vi "Valiadate Plugin Name.vi"(0 "Path":path, 5 "library name":string, 11 "error in (no error)":errorcluster) -> (4 "Valid Name?":bool, 15 "error out":errorcluster)   [LabVIEW 2021, in "Migrator.lvlib"]
uses:
  Migrator.lvlib
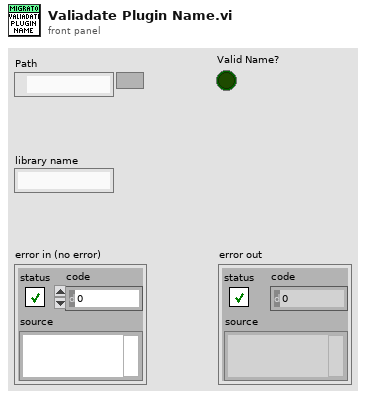
[diagram p1: front panel]
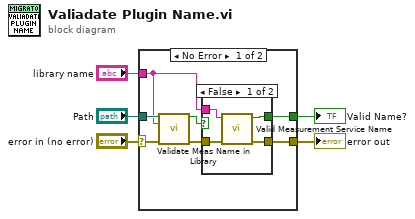
[diagram p0: block diagram]
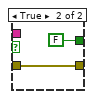
[diagram p2: hidden frame]
diagram:
  n1 = case shown="No Error" "error in (no error)" {
    selector: "error in (no error)" -> [w7 w19]
    tunnel: "Path" -> [w12 _]
    tunnel: "library name" -> [w9 _]
    tunnel: [w8 _] -> w2
    tunnel: [w6 w19] -> w1
    frame No Error {
      n2 = call "Validate Meas Name in Library.vi"("Path"=w12, "library name"=w9, "error in (no error)"=w7) -> ("found"=w11:bool, "error out"=w10:errorcluster)  [unwired: 11 in]
      n3 = case shown="False" w11 {
        tunnel: w10 -> [w15 w18]
        tunnel: w9 -> [w14 _]
        tunnel: [w13 FALSE ("valid name?")] -> w8
        tunnel: [w16 w18] -> w6
        frame False {
          n4 = call "Valid Measurement Service Name.vi"("error in"=w15, "requested plugin name"=w14) -> ("error out"=w16:errorcluster, "valid name?"=w13:bool)  [unwired: 8 in]
        }
        frame True {
        }
      }
    }
    frame Error {
    }
  }
  "error out" <- w1
  "Valid Name?" <- w2
